vi "Config Format.vi"(6 "Field Width (fixed)":u16(ring) items=["Variable", "Fixed", ""], 7 "Notation (floating)":u16(ring) items=["Floating", "Scientific", "Engineering"], 8 "error in":errorcluster, 9 "IEEE 488.2 (off)":bool, 10 "Labelling (on)":bool=TRUE, 11 "VISA resource name":refnum<visa-resource-name>) -> (0 "error out":errorcluster, 3 "VISA resource name out":refnum<visa-resource-name>)   [LabVIEW 2016, in "Andeen-Hagerling 2550.lvlib"]
doc: "This VI controls the format and numeric notation of results which are sent to serial or GPIB ports. Front panel results are not affected. Note that default parameter values correspond to the bridge default values and not the values assigned in <b>Default Instrument Setup.vi</b>."
uses:
  Andeen-Hagerling 2550.lvlib
panel:
  # "Format Parameters"
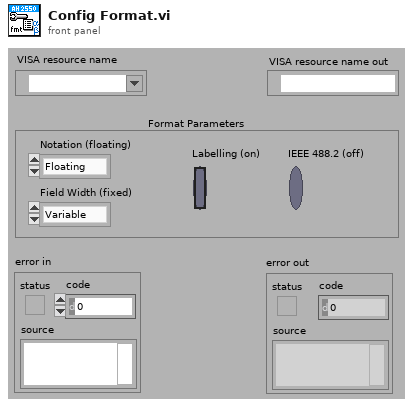
[diagram p1: front panel]
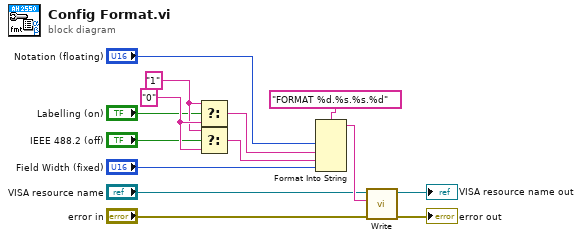
[diagram p0: block diagram]
diagram:
  w14 = "0"
  w13 = "1"
  n1 = Select(t=w13, s="Labelling (on)", f=w14) -> (s? t:f=w9:string)
  n2 = Select(t=w13, s="IEEE 488.2 (off)", f=w14) -> (s? t:f=w8:string)
  n3 = Format Into String(format string="FORMAT %d.%s.%s.%d", "Notation (floating)", w9, w8, "Field Width (fixed)") -> (resulting string=w12:string)  [unwired: 2 in, 1 out]
  n4 = call "Write.vi"("error in"="error in", "command"=w12, "VISA resource name"="VISA resource name") -> ("error out"=→"error out":errorcluster, "VISA resource name out"=→"VISA resource name out":refnum<visa-resource-name>)  [unwired: 7 in]
